vi "Proof Checksum.vi"(3 "Error In":errorcluster, 5 "Read Buffer":string) -> (0 "Error Out":errorcluster, 1 "Checksum OK?":bool, 2 "Response":string)   [LabVIEW 2016, in "KIT QV.lvlib"]
doc: "Proof checksum of instrument response."
uses:
  KIT QV.lvlib
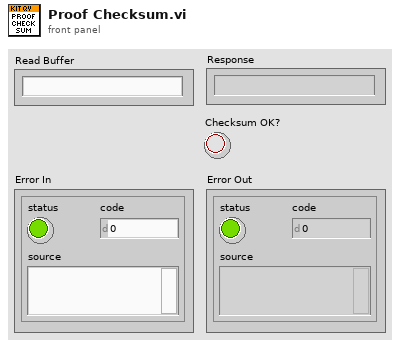
[diagram p1: front panel]
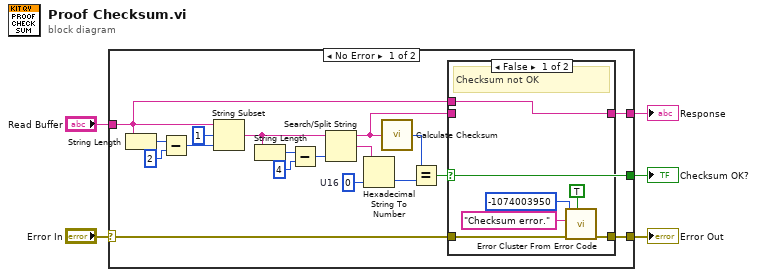
[diagram p0: block diagram]
diagram:
  n1 = case shown="No Error" "Error In" {
    selector: "Error In" -> [w11 w32]
    tunnel: "Read Buffer" -> [w6 w33]
    tunnel: [w9 _] -> w4
    tunnel: [w7 w33] -> w3
    tunnel: [w10 w32] -> w1
    frame No Error {
      w14 = u16 0  # U16
      n2 = String Length(string=w6) -> (length=w22:i32)
      n3 = Subtract(x=w22, y=2 ("offset (0)")) -> (x-y=w20:i32)
      n4 = String Subset(string=w6, offset (0)=1, length (rest)=w20) -> (substring=w17:string)
      n5 = String Length(string=w17) -> (length=w18:i32)
      n6 = Subtract(x=w18, y=4 ("offset (0)")) -> (x-y=w16:i32)
      n7 = Search/Split String(string=w17, offset (0)=w16) -> (substring before match=w8:string, match + rest of string=w15:string)  [unwired: 1 in, 1 out]
      n8 = Hexadecimal String To Number(string=w15, default (0uL)=w14) -> (number=w12:u16)  [unwired: 1 in, 1 out]
      n9 = call "Calculate Checksum.vi"("String in"=w8) -> ("Checksum"=w13:u16)
      n10 = Equal?(x=w13, y=w12) -> (x = y?=w9:bool)
      n11 = case shown="False" w9 {
        tunnel: w11 -> [w29 w30]
        tunnel: [w28 w30] -> w10
        tunnel: w8 -> [_ w31]
        tunnel: [w24 w31] -> w7
        tunnel: w6 -> [w24 _]
        frame False {
          # "Checksum not OK"
          n12 = call <vilib>:"Error Cluster From Error Code.vi"("show call chain? (False)"=TRUE, "error in (no error)"=w29, "error message (\"\")"="Checksum error." ("error message (\"\")"), "error code (0)"=-1074003950) -> ("error out"=w28:errorcluster)  [unwired: 5 in]
        }
        frame True {
          # "Checksum OK"
        }
      }
    }
    frame Error {
    }
  }
  "Response" <- w3
  "Checksum OK?" <- w4
  "Error Out" <- w1
